vi "Upload to Arduino.vi"() -> ()   [LabVIEW 2019]
panel:
  in  "OK Button":bool
  in  "File name":string
  in  "code":string
  in  "Packages":path
  in  "Java":path
  out "Output":string
  out "Error":string
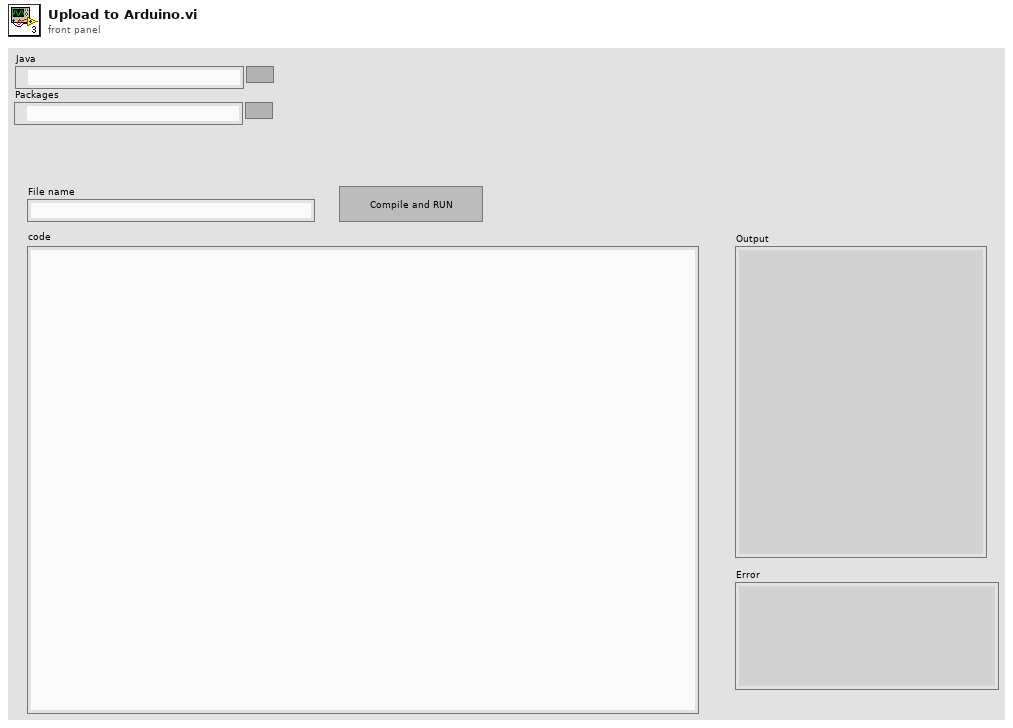
[diagram p1: front panel]
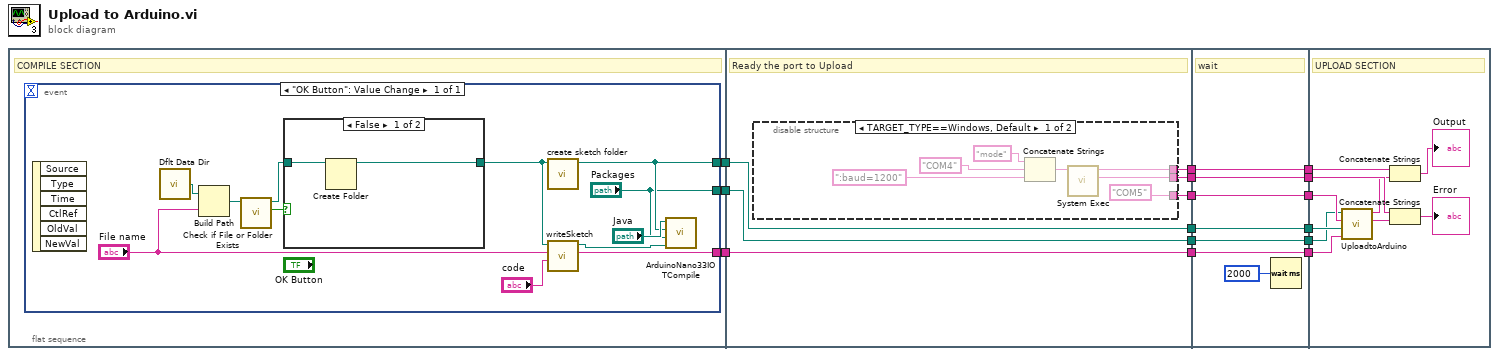
[diagram p0: block diagram]
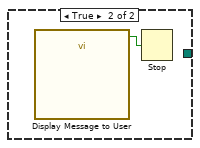
[diagram p2: hidden frame]
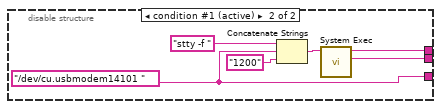
[diagram p3: hidden frame]
diagram:
  n1 = flat-sequence {
    tunnel: [w18] -> w7
    tunnel: [w17] -> w6
    tunnel: [w16] -> w1
    tunnel: [w34] -> w15
    tunnel: [w35] -> w12
    tunnel: [w36] -> w11
    tunnel: [w39] -> w8
    tunnel: w7 -> [w39]
    tunnel: w6 -> [w38]
    tunnel: [w38] -> w5
    tunnel: [w37] -> w2
    tunnel: w1 -> [w37]
    tunnel: w15 -> [w58]
    tunnel: [w58] -> w14
    tunnel: [w57] -> w13
    tunnel: w12 -> [w57]
    tunnel: w11 -> [w56]
    tunnel: [w56] -> w10
    tunnel: [w55] -> w9
    tunnel: w8 -> [w55]
    tunnel: w5 -> [w54]
    tunnel: [w54] -> w4
    tunnel: [w53] -> w3
    tunnel: w2 -> [w53]
    tunnel: w14 -> [w62]
    tunnel: w13 -> [w69]
    tunnel: w10 -> [w66]
    tunnel: w9 -> [w61]
    tunnel: w4 -> [w63]
    tunnel: w3 -> [w60]
    frame #0 {
      # "COMPILE SECTION"
      n2 = event shown="[0] \"OK Button\": Value Change" {
        selector: _ -> [_]
        dyn-events: _ -> [_]
        timeout: _ -> [_]
        tunnel: [w28] -> w18
        tunnel: [w25] -> w17
        tunnel: ["Packages"] -> w16
        event "OK Button": Value Change {
          n3 = event-data() -> ()  [unwired: 1 in, 6 out]
          n4 = call <vilib>:"Dflt Data Dir.vi"() -> ("App:Default Data Directory"=w27:path)
          n5 = Build Path(base path=w27, name or relative path="File name") -> (appended path=w23:path)
          n6 = call <vilib>:"Check if File or Folder Exists.vi"("path"=w23) -> ("file or folder exists?"=w24:bool, "dup path"=w21:path)  [unwired: 8 in, 1 out]
          n7 = case shown="False" w24 {
            tunnel: [w32 _] -> w22
            tunnel: w21 -> [w31 _]
            frame False {
              n8 = Create Folder(path (use dialog)=w31) -> (created path=w32:path)  [unwired: 2 in, 2 out]
            }
            frame True {
              n9 = call "Display Message to User"() -> ("OK"=w33:bool)  [unwired: 10 in, 1 out]
              n10 = Stop(stop? (T)=w33) -> ()
            }
          }
          n11 = call "create sketch folder.vi"("path to ino folder"=w22) -> ("path to sketch folder"=w28:path)  [unwired: 10 in]
          n12 = call "writeSketch.vi"("Code"="code", "File name"="File name", "path to ino folder"=w22) -> ("Sketch.ino"=w25:string, "path to ino file"=w29:path)  [unwired: 7 in]
          n13 = call "ArduinoNano33IOTCompile.vi"("ino file"=w29, "Packages"="Packages", "bin location to upload"=w28, "Java"="Java") -> ()  [unwired: 6 in, 2 out]
        }
      }
    }
    frame #1 {
      # "Ready the port to Upload"
      n14 = disable-structure shown="TARGET_TYPE==Windows, Default" {
        disable-tunnel: [w42 w49] -> w36
        disable-tunnel: [w41 w48] -> w35
        disable-tunnel: ["COM5" ("string") w47] -> w34
        frame condition #0 {
          n15 = Concatenate Strings("mode" ("string"), "COM4" ("string"), ":baud=1200" ("string")) -> (w46:string)
          n16 = call <vilib>:"System Exec.vi"("command line"=w46) -> ("standard error"=w41:string, "standard output"=w42:string)  [unwired: 7 in, 2 out]
        }
        frame condition #1 (active) {
          w47 = "/dev/cu.usbmodem14101 " ("string")
          n17 = Concatenate Strings("stty -f " ("string"), w47, "1200" ("string")) -> (w52:string)
          n18 = call <vilib>:"System Exec.vi"("command line"=w52) -> ("standard error"=w48:string, "standard output"=w49:string)  [unwired: 7 in, 2 out]
        }
      }
    }
    frame #2 {
      # "wait"
      n19 = Wait (ms)(milliseconds to wait=u32 2000) -> ()  [unwired: 1 out]
    }
    frame #3 {
      # "UPLOAD SECTION"
      n20 = call "UploadtoArduino.vi"("Sketch.ino"=w63, "path to sketch folder"=w61, "serial port"=w62, "path to bossac"=w60) -> ("standard error"=w68:string, "standard output"=w65:string)  [unwired: 6 in]
      n21 = Concatenate Strings(w66, w65) -> (→"Output":string)
      n22 = Concatenate Strings(w69, w68) -> (→"Error":string)
    }
  }
